vi "log analysis_gps.vi"() -> ()   [LabVIEW 2019] (continued)
normal 2 28.000000 0 0\trobot status\t224.454094\t106.289385\t8.223600\t-0.397359\t-0.581660\t162.070922\t0.000000\t0.000000\n\t\n15:40:00.3\tlog_raw\tgps_raw\t\tsystem status\tnormal 2 28.000000 0 0\trobot status\t224.454354\t106.289109\t8.223500\t-0.396354\t-0.583432\t162.070544\t0.000000\t0.000000\n\t\n15:40:00.8\tlog_raw\tgps_raw\t#INSPVAXA,USB3,0,49.0,FINESTEERING,2107,283218.850,02000000,471d,15824;INS_ALIGNMENT_COMPLETE,INS_RTKFIXED,37.37108791456,126.72336907619,8.2236,22.3000,0.0037,0.0083,-0.0011,-0.397325323,-0.588631877,287.932091771,0.2122,0.1575,0.2639,0.0344,0.0343,0.0312,0.0792,0.0802,5.0844,0f000005,0*75bb9db3\n\tsystem status\tnormal 2 28.000000 0 0\trobot status\t224.455009\t106.288943\t8.223600\t-0.397325\t-0.588632\t162.067908\t0.000000\t0.000000\n\t\n15:40:01.3\tlog_raw\tgps_raw\t#INSPVAXA,USB3,0,48.5,FINESTEERING,2107,283219.350,02000000,471d,15824;INS_ALIGNMENT_COMPLETE,INS_RTKFIXED,37.37108791216,126.72336907891,8.2235,22.3000,0.0033,0.0082,-0.0011,-0.397206354,-0.592415954,287.932797733,0.2122,0.1575,0.2639,0.0344,0.0343,0.0312,0.0792,0.0802,5.0858,0f000005,0*61ec993c\n\tsystem status\tnormal 2 28.000000 0 0\trobot status\t224.455250\t106.288677\t8.223500\t-0.397206\t-0.592416\t162.067202\t0.000000\t0.000000\n\t\n15:40:01.8\tlog_raw\tgps_raw\t#DUALANTENNAHEADINGA,USB3,0,48.5,FINESTEERING,2107,283219.800,02000000,d426,15824;INSUFFICIENT_OBS,NONE,-1.000000000,0.000000000,0.000000000,0.0,0.000000000,0.000000000,\"631T\",12,4,4,3,04,00,20,03*1f4b872e\n\tsystem status\tnormal 2 28.000000 0 0\trobot status\t224.455582\t106.288430\t8.223100\t-0.398043\t-0.597040\t162.064293\t0.000000\t0.000000\n\t\n15:40:02.3\tlog_raw\tgps_raw\t#INSPVAXA,USB3,0,49.5,FINESTEERING,2107,283220.350,02000000,471d,15824;INS_ALIGNMENT_COMPLETE,INS_RTKFIXED,37.37108790624,126.72336908505,8.2229,22.3000,0.0022,0.0079,-0.0019,-0.399821313,-0.599696922,287.937754794,0.2122,0.1575,0.2639,0.0344,0.0343,0.0312,0.0792,0.0802,5.0871,0f000005,0*02520bc5\n\tsystem status\tnormal 2 28.000000 0 0\trobot status\t224.455794\t106.288020\t8.222900\t-0.399821\t-0.599697\t162.062245\t0.000000\t0.000000\n\t\n15:40:02.8\tlog_raw\tgps_raw\t#DUALANTENNAHEADINGA,USB3,0,49.5,FINESTEERING,2107,283220.800,02000000,d426,15824;INSUFFICIENT_OBS,NONE,-1.000000000,0.000000000,0.000000000,0.0,0.000000000,0.000000000,\"631T\",14,4,4,3,04,00,20,03*89ffa4d7\n\tsystem status\tnormal 2 28.000000 0 0\trobot status\t224.456145\t106.287761\t8.222900\t-0.400058\t-0.601408\t162.059931\t0.000000\t0.000000\n\t\n15:40:03.3\tlog_raw\tgps_raw\t#INSPVAXA,USB3,0,50.0,FINESTEERING,2107,283221.350,02000000,471d,15824;INS_ALIGNMENT_COMPLETE,INS_RTKFIXED,37.37108790285,126.72336908925,8.2228,22.3000,0.0035,0.0061,-0.0019,-0.399017543,-0.601198983,287.941471827,0.2122,0.1575,0.2639,0.0344,0.0343,0.0312,0.0792,0.0802,5.0886,0f000005,0*62ae3a3c\n\tsystem status\tnormal 2 28.000000 0 0\trobot status\t224.456166\t106.287643\t8.222800\t-0.399018\t-0.601199\t162.058528\t0.000000\t0.000000\n\t\n15:40:03.8\tlog_raw\tgps_raw\t#DUALANTENNAHEADINGA,USB3,0,50.0,FINESTEERING,2107,283221.800,02000000,d426,15824;INSUFFICIENT_OBS,NONE,-1.000000000,0.000000000,0.000000000,0.0,0.000000000,0.000000000,\"631T\",15,4,4,3,04,00,20,03*47e08abb\n\tsystem status\tnormal 2 28.000000 0 0\trobot status\t224.456082\t106.288102\t8.222400\t-0.398407\t-0.602014\t162.056223\t0.000000\t0.000000\n\t\n15:40:04.3\tlog_raw\tgps_raw\t#INSPVAXA,USB3,0,45.5,FINESTEERING,2107,283222.350,02000000,471d,15824;INS_ALIGNMENT_COMPLETE,INS_RTKFIXED,37.37108790796,126.72336908471,8.2224,22.3000,0.0048,0.0047,-0.0019,-0.398683572,-0.604525422,287.944164472,0.2123,0.1575,0.2638,0.0344,0.0343,0.0312,0.0792,0.0802,5.0901,0f000005,0*5070a156\n\tsystem status\tnormal 2 28.000000 0 0\trobot status\t224.455764\t106.288211\t8.222400\t-0.398684\t-0.604525\t162.055836\t0.000000\t0.000000\n\t\n15:40:04.8\tlog_raw\tgps_raw\t#DUALANTENNAHEADINGA,USB3,0,45.5,FINESTEERING,2107,283222.800,02000000,d426,15824;INSUFFICIENT_OBS,NONE,-1.000000000,0.000000000,0.000000000,0.0,0.000000000,0.000000000,\"631T\",14,4,4,3,04,00,20,03*8ce94816\n\tsystem status\tnormal 2 28.000000 0 0\trobot status\t224.455489\t106.288239\t8.222400\t-0.397979\t-0.605286\t162.052954\t0.000000\t0.000000\n\t\n15:40:05.3\tlog_raw\tgps_raw\t#INSPVAXA,USB3,0,50.0,FINESTEERING,2107,283223.350,02000000,471d,15824;INS_ALIGNMENT_COMPLETE,INS_RTKFIXED,37.37108790821,126.72336907660,8.2226,22.3000,0.0055,0.0030,-0.0018,-0.398800774,-0.606505226,287.948554602,0.2123,0.1575,0.2638,0.0344,0.0343,0.0312,0.0792,0.0802,5.0917,0f000005,0*2b7dac3f\n\tsystem status\tnormal 2 28.000000 0 0\trobot status\t224.455045\t106.288238\t8.222600\t-0.398801\t-0.606505\t162.051445\t0.000000\t0.000000\n\t\n15:40:05.8\tlog_raw\tgps_raw\t\tsystem status\tnormal 2 28.000000 0 0\trobot status\t224.454616\t106.288408\t8.223000\t-0.399540\t-0.605602\t162.051000\t0.000000\t0.000000\n\t\n15:40:06.3\tlog_raw\tgps_raw\t#DUALANTENNAHEADINGA,USB3,0,49.5,FINESTEERING,2107,283224.300,02000000,d426,15824;INSUFFICIENT_OBS,NONE,-1.000000000,0.000000000,0.000000000,0.0,0.000000000,0.000000000,\"631T\",16,4,4,3,04,00,20,03*04689537\n\tsystem status\tnormal 2 28.000000 0 0\trobot status\t224.454250\t106.288382\t8.223000\t-0.399365\t-0.605451\t162.052103\t0.000000\t0.000000\n\t\n15:40:06.8\tlog_raw\tgps_raw\t#INSPVAXA,USB3,0,49.5,FINESTEERING,2107,283224.850,02000000,471d,15824;INS_ALIGNMENT_COMPLETE,INS_RTKFIXED,37.37108790871,126.72336906996,8.2222,22.3000,0.0045,0.0021,-0.0033,-0.398675673,-0.605186622,287.948531011,0.2123,0.1575,0.2638,0.0344,0.0343,0.0312,0.0792,0.0802,5.0933,0f000005,0*5d419d28\n\tsystem status\tnormal 2 28.000000 0 0\trobot status\t224.454457\t106.288294\t8.222200\t-0.398676\t-0.605187\t162.051469\t0.000000\t0.000000\n\t\n15:40:07.3\tlog_raw\tgps_raw\t#INSPVAXA,USB3,0,47.0,FINESTEERING,2107,283225.350,02000000,471d,15824;INS_ALIGNMENT_COMPLETE,INS_RTKFIXED,37.37108790579,126.72336906833,8.2219,22.3000,0.0039,0.0019,-0.0038,-0.399713651,-0.605242342,287.947949852,0.2123,0.1575,0.2638,0.0344,0.0343,0.0312,0.0792,0.0802,5.0949,0f000005,0*a40dd195\n\tsystem status\tnormal 2 28.000000 0 0\trobot status\t224.454313\t106.287970\t8.221900\t-0.399714\t-0.605242\t162.052050\t0.000000\t0.000000\n\t\n15:40:07.8\tlog_raw\tgps_raw\t#INSPVAXA,USB3,0,47.0,FINESTEERING,2107,283225.850,02000000,471d,15824;INS_ALIGNMENT_COMPLETE,INS_RTKFIXED,37.37108794475,126.72336891478,8.2224,22.3000,0.0658,-0.1833,-0.0010,-0.392923625,-0.435798491,288.066022775,0.2123,0.1575,0.2638,0.0344,0.0343,0.0312,0.0792,0.0802,5.0949,0f000005,0*2ff36e63\n\tsystem status\tnormal 2 27.900000 0 0\trobot status\t224.440712\t106.292294\t8.222400\t-0.392924\t-0.435798\t161.933977\t0.180000\t0.055000\n\t\n15:40:08.3\tlog_raw\tgps_raw\t#INSPVAXA,USB3,0,49.0,FINESTEERING,2107,283226.350,02000000,471d,15824;INS_ALIGNMENT_COMPLETE,INS_RTKFIXED,37.37108844765,126.72336703725,8.2202,22.3000,0.1175,-0.3192,-0.0049,-0.452699232,-0.802169824,288.131784608,0.2162,0.1626,0.2698,0.0571,0.0479,0.0400,0.0831,0.0841,5.0965,0f000001,0*8912b163\n\tsystem status\tnormal 2 28.000000 0 0\trobot status\t224.274403\t106.348113\t8.220200\t-0.452699\t-0.802170\t161.868215\t0.327000\t-0.008000\n\t\n15:40:08.8\tlog_raw\tgps_raw\t\tsystem status\tnormal 2 28.000000 0 0\trobot status\t224.153734\t106.388805\t8.217000\t-0.710423\t-0.963431\t161.777362\t0.275000\t0.048000\n\t\n15:40:09.3\tlog_raw\tgps_raw\t#INSPVAXA,USB3,0,48.5,FINESTEERING,2107,283227.350,02000000,471d,15824;INS_ALIGNMENT_COMPLETE,INS_RTKFIXED,37.37108931483,126.72336395391,8.2149,22.3000,0.1129,-0.2937,-0.0022,-0.567222074,-1.168347253,288.238962529,0.2212,0.1749,0.2808,0.0651,0.0592,0.0471,0.0869,0.0878,5.0924,0f000001,0*8f246b52\n\tsystem status\tnormal 2 28.000000 0 0\trobot status\t224.001286\t106.444364\t8.214900\t-0.567222\t-1.168347\t161.761037\t0.292000\t0.057000\n\t\n15:40:09.8\tlog_raw\tgps_raw\t#INSPVAXA,USB3,0,48.5,FINESTEERING,2107,283227.850,02000000,471d,15824;INS_ALIGNMENT_COMPLETE,INS_RTKFIXED,37.37108976815,126.72336241064,8.2129,22.3000,0.1012,-0.2894,0.0009,-0.427491703,-1.215964317,288.177638677,0.2212,0.1749,0.2808,0.0651,0.0592,0.0471,0.0869,0.0878,5.0924,0f000001,0*ddfdf890\n\tsystem status\tnormal 2 27.900000 0 0\trobot status\t223.864586\t106.494679\t8.212900\t-0.427492\t-1.215964\t161.822361\t0.383000\t-0.102000\n\t\n15:40:10.3\tlog_raw\tgps_raw\t#INSPVAXA,USB3,0,43.5,FINESTEERING,2107,283228.350,02000000,471d,15824;INS_ALIGNMENT_COMPLETE,INS_RTKFIXED,37.37109022271,126.72336087108,8.2100,22.3000,0.0996,-0.2735,0.0003,-0.409798448,-1.329111694,287.820965193,0.2393,0.1944,0.2974,0.0761,0.0698,0.0531,0.0903,0.0914,5.0788,0f000001,0*ba2a3ea8\n\tsystem status\tnormal 2 27.900000 0 0\trobot status\t223.728214\t106.545132\t8.210000\t-0.409798\t-1.329112\t162.179035\t0.286000\t0.039000\n\t\n15:40:10.8\tlog_raw\tgps_raw\t#INSPVAXA,USB3,0,43.5,FINESTEERING,2107,283228.850,02000000,471d,15824;INS_ALIGNMENT_COMPLETE,INS_RTKFIXED,37.37109066362,126.72335936248,8.2065,22.3000,0.0986,-0.2652,0.0020,-0.598740198,-1.345095429,287.386151451,0.2393,0.1944,0.2974,0.0761,0.0698,0.0531,0.0903,0.0914,5.0788,0f000001,0*2e7dd81d\n\tsystem status\tnormal 2 27.900000 0 0\trobot status\t223.594584\t106.594070\t8.206500\t-0.598740\t-1.345095\t162.613849\t0.240000\t0.109000\n\t\n15:40:11.3\tlog_raw\tgps_raw\t#INSPVAXA,USB3,0,48.5,FINESTEERING,2107,283229.350,02000000,471d,15824;INS_ALIGNMENT_COMPLETE,INS_RTKFIXED,37.37109112291,126.72335786047,8.2034,22.3000,0.1037,-0.2722,0.0059,-0.580011682,-1.182180858,286.853066758,0.2680,0.2186,0.3192,0.0865,0.0782,0.0582,0.0931,0.0946,5.0540,0f000001,0*9b5ccdcf\n\tsystem status\tnormal 2 27.800000 0 0\trobot status\t223.461539\t106.645047\t8.203400\t-0.580012\t-1.182181\t163.146933\t0.284000\t0.047000\n\t\n15:40:11.8\tlog_raw\tgps_raw\t#INSPVAXA,USB3,0,48.5,FINESTEERING,2107,283229.850,02000000,471d,15824;INS_ALIGNMENT_COMPLETE,INS_RTKFIXED,37.37109159656,126.72335634766,8.2007,22.3000,0.0997,-0.2660,0.0048,-0.505114639,-1.253978500,286.329147717,0.2680,0.2186,0.3192,0.0865,0.0782,0.0582,0.0931,0.0946,5.0540,0f000001,0*b8c54619\n\tsystem status\tnormal 2 27.800000 0 0\trobot status\t223.327537\t106.697619\t8.200700\t-0.505115\t-1.253979\t163.670852\t0.201000\t0.152000\n\t\n15:40:12.3\tlog_raw\tgps_raw\t\tsystem status\tnormal 2 27.800000 0 0\trobot status\t223.205787\t106.745862\t8.197500\t-0.502623\t-1.292688\t164.218848\t0.298000\t0.019000\n\t\n15:40:12.8\tlog_raw\tgps_raw\t#INSPVAXA,USB3,0,48.5,FINESTEERING,2107,283230.850,02000000,471d,15824;INS_ALIGNMENT_COMPLETE,INS_RTKFIXED,37.37109255379,126.72335333433,8.1922,22.3000,0.1139,-0.2722,-0.0264,-0.549844601,-1.243677147,285.192352879,0.3030,0.2423,0.3452,0.0951,0.0845,0.0626,0.0951,0.0973,5.0218,0f000001,0*4712ada1\n\tsystem status\tnormal 2 27.700000 0 0\trobot status\t223.060621\t106.803864\t8.192200\t-0.549845\t-1.243677\t164.807647\t0.237000\t0.112000\n\t\n15:40:13.3\tlog_raw\tgps_raw\t\tsystem status\tnormal 2 27.800000 0 0\trobot status\t222.939771\t106.853141\t8.188200\t-0.588387\t-1.223015\t165.124564\t0.226000\t0.121000\n\t\n15:40:13.8\tlog_raw\tgps_raw\t#INSPVAXA,USB3,0,47.5,FINESTEERING,2107,283231.850,02000000,471d,15824;INS_ALIGNMENT_COMPLETE,INS_RTKFIXED,37.37109356016,126.72335031478,8.1824,22.3000,0.1080,-0.2773,-0.0065,-0.427440692,-1.278596031,284.403841092,0.3386,0.2620,0.3738,0.1014,0.0883,0.0663,0.0962,0.0993,4.9874,0f000001,0*03e37570\n\tsystem status\tnormal 2 27.900000 0 0\trobot status\t222.793154\t106.915562\t8.182400\t-0.427441\t-1.278596\t165.596159\t0.216000\t0.140000\n\t\n15:40:14.3\tlog_raw\tgps_raw\t\tsystem status\tnormal 2 27.900000 0 0\trobot status\t222.674508\t106.965363\t8.178200\t-0.397587\t-1.349561\t165.862378\t0.359000\t-0.071000\n\t\n15:40:14.8\tlog_raw\tgps_raw\t\tsystem status\tnormal 2 27.900000 0 0\trobot status\t222.542928\t107.019957\t8.172800\t-0.416047\t-1.243660\t166.159650\t0.279000\t0.039000\n\t\n15:40:15.3\tlog_raw\tgps_raw\t#INSPVAXA,USB3,0,48.5,FINESTEERING,2107,283233.350,02000000,471d,15824;INS_ALIGNMENT_COMPLETE,INS_RTKFIXED,37.37109506136,126.72334582781,8.1673,22.3000,0.1059,-0.2882,-0.0129,-0.399188016,-1.308966160,283.569134485,0.3953,0.2852,0.4320,0.1083,0.0909,0.0717,0.0969,0.1016,4.9362,0f000001,0*c0c0ad69\n\tsystem status\tnormal 2 27.900000 0 0\trobot status\t222.395706\t107.082183\t8.167300\t-0.399188\t-1.308966\t166.430866\t0.280000\t0.051000\n\t\n15:40:15.8\tlog_raw\tgps_raw\t#INSPVAXA,USB3,0,48.5,FINESTEERING,2107,283233.850,02000000,471d,15824;INS_ALIGNMENT_COMPLETE,INS_RTKFIXED,37.37109557748,126.72334434749,8.1612,22.3000,0.1020,-0.2689,-0.0118,-0.288207427,-1.260427493,283.382499321,0.3953,0.2852,0.4320,0.1083,0.0909,0.0717,0.0969,0.1016,4.9362,0f000001,0*9cae95f0\n\tsystem status\tnormal 2 27.900000 0 0\trobot status\t222.264581\t107.139468\t8.161200\t-0.288207\t-1.260427\t166.617501\t0.269000\t0.054000\n\t\n15:40:16.3\tlog_raw\tgps_raw\t#INSPVAXA,USB3,0,40.5,FINESTEERING,2107,283234.350,02000000,471d,15824;INS_ALIGNMENT_COMPLETE,INS_RTKFIXED,37.37109597071,126.72334335857,8.1556,22.3000,0.0926,-0.1801,-0.0168,-0.385399344,-0.992179167,283.170226692,0.4136,0.2904,0.4588,0.1097,0.0911,0.0735,0.0969,0.1021,4.9239,0f000001,0*8e2cf425\n\tsystem status\tnormal 2 27.900000 0 0\trobot status\t222.176984\t107.183113\t8.155600\t-0.385399\t-0.992179\t166.829773\t0.175000\t0.049000\n\t\n15:40:16.8\tlog_raw\tgps_raw\t\tsystem status\tnormal 2 27.900000 0 0\trobot status\t222.041325\t107.237168\t8.148500\t-0.223084\t-1.273652\t166.883018\t0.182000\t0.108000\n\t\n15:40:17.3\tlog_raw\tgps_raw\t#INSPVAXA,USB3,0,44.5,FINESTEERING,2107,283235.350,02000000,471d,15824;INS_ALIGNMENT_COMPLETE,INS_RTKFIXED,37.37109700062,126.72334017325,8.1414,22.3000,0.1228,-0.2164,-0.0234,-0.044307272,-1.163346566,282.981780278,0.4261,0.2932,0.4825,0.1104,0.0912,0.0747,0.0969,0.1023,4.9187,0f000001,0*f944742e\n\tsystem status\tnormal 2 27.900000 0 0\trobot status\t221.894834\t107.297424\t8.141400\t-0.044307\t-1.163347\t167.018220\t0.186000\t0.129000\n\t\n15:40:17.8\tlog_raw\tgps_raw\t#INSPVAXA,USB3,0,44.5,FINESTEERING,2107,283235.850,02000000,471d,15824;INS_ALIGNMENT_COMPLETE,INS_RTKFIXED,37.37109748848,126.72333864124,8.1345,22.3000,0.1343,-0.2501,-0.0261,0.047074074,-1.173722020,282.896627938,0.4261,0.2932,0.4825,0.1104,0.0912,0.0747,0.0969,0.1023,4.9187,0f000001,0*d201ba2d\n\tsystem status\tnormal 2 27.900000 0 0\trobot status\t221.759131\t107.351573\t8.134500\t0.047074\t-1.173722\t167.103372\t0.376000\t-0.123000\n\t\n15:40:18.3\tlog_raw\tgps_raw\t#INSPVAXA,USB3,0,49.0,FINESTEERING,2107,283236.350,02000000,471d,15824;INS_ALIGNMENT_COMPLETE,INS_RTKFIXED,37.37109796118,126.72333710973,8.1282,22.3000,0.1356,-0.2699,-0.0252,0.117707289,-1.086574547,282.783735366,0.4343,0.2946,0.5028,0.1112,0.0912,0.0756,0.0969,0.1025,4.9173,0f000001,0*2a8403f7\n\tsystem status\tnormal 2 27.900000 0 0\trobot status\t221.623472\t107.404039\t8.128200\t0.117707\t-1.086575\t167.216265\t0.368000\t-0.094000\n\t\n15:40:18.8\tlog_raw\tgps_raw\t#INSPVAXA,USB3,0,49.0,FINESTEERING,2107,283236.850,02000000,471d,15824;INS_ALIGNMENT_COMPLETE,INS_RTKFIXED,37.37109843766,126.72333556115,8.1224,22.3000,0.1364,-0.2752,-0.0170,0.206554754,-1.115785286,282.668706587,0.4343,0.2946,0.5028,0.1112,0.0912,0.0756,0.0969,0.1025,4.9173,0f000001,0*f32b757d\n\tsystem status\tnormal 2 27.900000 0 0\trobot status\t221.486302\t107.456924\t8.122400\t0.206555\t-1.115785\t167.331293\t0.349000\t-0.069000\n\t\n15:40:19.3\tlog_raw\tgps_raw\t#INSPVAXA,USB3,0,50.0,FINESTEERING,2107,283237.350,02000000,471d,15824;INS_ALIGNMENT_COMPLETE,INS_RTKFIXED,37.37109889709,126.72333402852,8.1172,22.3000,0.1302,-0.2622,-0.0159,0.272964655,-0.969484685,282.581344879,0.4398,0.2952,0.5196,0.1116,0.0914,0.0761,0.0969,0.1026,4.9185,0f000001,0*477c8ced\n\tsystem status\tnormal 2 27.900000 0 0\trobot status\t221.350544\t107.507918\t8.117200\t0.272965\t-0.969485\t167.418655\t0.348000\t-0.074000\n\t\n15:40:19.8\tlog_raw\tgps_raw\t#INSPVAXA,USB3,0,50.0,FINESTEERING,2107,283237.850,02000000,471d,15824;INS_ALIGNMENT_COMPLETE,INS_RTKFIXED,37.37109934536,126.72333248224,8.1121,22.3000,0.1280,-0.2768,-0.0138,0.258054665,-1.050370160,282.484517090,0.4398,0.2952,0.5196,0.1116,0.0914,0.0761,0.0969,0.1026,4.9185,0f000001,0*cd2f787f\n\tsystem status\tnormal 2 27.900000 0 0\trobot status\t221.213577\t107.557672\t8.112100\t0.258055\t-1.050370\t167.515483\t0.336000\t-0.058000\n\t\n15:40:20.3\tlog_raw\tgps_raw\t#INSPVAXA,USB3,0,51.5,FINESTEERING,2107,283238.350,02000000,471d,15824;INS_ALIGNMENT_COMPLETE,INS_RTKFIXED,37.37109977982,126.72333093578,8.1070,22.3000,0.1223,-0.2761,-0.0142,0.234355283,-1.035161651,282.464995705,0.4436,0.2955,0.5329,0.1118,0.0916,0.0764,0.0970,0.1026,4.9197,0f000001,0*b2aac9f1\n\tsystem status\tnormal 2 27.900000 0 0\trobot status\t221.076594\t107.605894\t8.107000\t0.234355\t-1.035162\t167.535004\t0.373000\t-0.110000\n\t\n15:40:20.8\tlog_raw\tgps_raw\t#INSPVAXA,USB3,0,51.5,FINESTEERING,2107,283238.850,02000000,471d,15824;INS_ALIGNMENT_COMPLETE,INS_RTKFIXED,37.37110022418,126.72332937535,8.1011,22.3000,0.1168,-0.2700,-0.0206,0.387659618,-1.151934969,282.487408850,0.4436,0.2955,0.5329,0.1118,0.0916,0.0764,0.0970,0.1026,4.9197,0f000001,0*91317f18\n\tsystem status\tnormal 2 28.000000 0 0\trobot status\t220.938374\t107.655215\t8.101100\t0.387660\t-1.151935\t167.512591\t0.298000\t-0.003000\n\t\n15:40:21.3\tlog_raw\tgps_raw\t#INSPVAXA,USB3,0,49.0,FINESTEERING,2107,283239.350,02000000,471d,15824;INS_ALIGNMENT_COMPLETE,INS_RTKFIXED,37.37110063479,126.72332783214,8.0954,22.3000,0.1184,-0.2911,-0.0146,0.524963643,-1.181982568,282.530354498,0.4459,0.2956,0.5431,0.1123,0.0918,0.0765,0.0970,0.1026,4.9196,0f000001,0*aac06e63\n\tsystem status\tnormal 2 27.900000 0 0\trobot status\t220.801679\t107.700790\t8.095400\t0.524964\t-1.181983\t167.469646\t0.299000\t0.005000\n\t\n15:40:21.8\tlog_raw\tgps_raw\t#INSPVAXA,USB3,0,49.0,FINESTEERING,2107,283239.850,02000000,471d,15824;INS_ALIGNMENT_COMPLETE,INS_RTKFIXED,37.37110101931,126.72332626888,8.0896,22.3000,0.1173,-0.2983,-0.0228,0.347504334,-1.218326130,282.608811447,0.4459,0.2956,0.5431,0.1123,0.0918,0.0765,0.0970,0.1026,4.9196,0f000001,0*aaab564a\n\tsystem status\tnormal 2 27.900000 0 0\trobot status\t220.663208\t107.743470\t8.089600\t0.347504\t-1.218326\t167.391189\t0.313000\t-0.016000\n\t\n15:40:22.3\tlog_raw\tgps_raw\t#INSPVAXA,USB3,0,49.5,FINESTEERING,2107,283240.350,02000000,471d,15824;INS_ALIGNMENT_COMPLETE,INS_RTKFIXED,37.37110139226,126.72332471479,8.0839,22.3000,0.1052,-0.2558,-0.0218,0.111794667,-1.199195640,282.711507437,0.4475,0.2957,0.5507,0.1121,0.0921,0.0765,0.0971,0.1026,4.9179,0f000001,0*067ad1f3\n\tsystem status\tnormal 2 28.000000 0 0\trobot status\t220.525549\t107.784865\t8.083900\t0.111795\t-1.199196\t167.288493\t0.283000\t-0.006000\n\t\n15:40:22.8\tlog_raw\tgps_raw\t#INSPVAXA,USB3,0,49.5,FINESTEERING,2107,283240.850,02000000,471d,15824;INS_ALIGNMENT_COMPLETE,INS_RTKFIXED,37.37110178506,126.72332315971,8.0792,22.3000,0.1224,-0.2728,-0.0239,0.192223977,-1.143692824,282.808782455,0.4475,0.2957,0.5507,0.1121,0.0921,0.0765,0.0971,0.1026,4.9179,0f000001,0*4c669a89\n\tsystem status\tnormal 2 27.900000 0 0\trobot status\t220.387802\t107.828463\t8.079200\t0.192224\t-1.143693\t167.191218\t0.304000\t-0.009000\n\t\n15:40:23.3\tlog_raw\tgps_raw\t#INSPVAXA,USB3,0,46.0,FINESTEERING,2107,283241.350,02000000,471d,15824;INS_ALIGNMENT_COMPLETE,INS_RTKFIXED,37.37110216671,126.72332169027,8.0740,22.3000,0.1256,-0.2749,-0.0357,0.303484738,-0.991943095,282.906858014,0.4483,0.2959,0.5565,0.1130,0.0923,0.0766,0.0971,0.1026,4.9153,0f000001,0*4b7c655e\n\tsystem status\tnormal 2 27.900000 0 0\trobot status\t220.257642\t107.870824\t8.074000\t0.303485\t-0.991943\t167.093142\t0.302000\t-0.011000\n\t\n15:40:23.8\tlog_raw\tgps_raw\t\tsystem status\tnormal 2 28.000000 0 0\trobot status\t220.122992\t107.913992\t8.068800\t0.222586\t-0.858858\t166.913815\t0.296000\t-0.018000\n\t\n15:40:24.3\tlog_raw\tgps_raw\t#INSPVAXA,USB3,0,49.5,FINESTEERING,2107,283242.350,02000000,471d,15824;INS_ALIGNMENT_COMPLETE,INS_RTKFIXED,37.37110294523,126.72331868826,8.0634,22.3000,0.1292,-0.2803,-0.0380,0.123672513,-0.689289621,283.242371954,0.4492,0.2961,0.5604,0.1137,0.0926,0.0766,0.0971,0.1026,4.9113,0f000001,0*f9b22440\n\tsystem status\tnormal 2 27.900000 0 0\trobot status\t219.991729\t107.957235\t8.063400\t0.123673\t-0.689290\t166.757628\t0.298000\t-0.030000\n\t\n15:40:24.8\tlog_raw\tgps_raw\t#INSPVAXA,USB3,0,49.5,FINESTEERING,2107,283242.850,02000000,471d,15824;INS_ALIGNMENT_COMPLETE,INS_RTKFIXED,37.37110335770,126.72331719520,8.0593,22.3000,0.1255,-0.2698,-0.0380,0.121355626,-0.605377000,283.439898811,0.4492,0.2961,0.5604,0.1137,0.0926,0.0766,0.0971,0.1026,4.9113,0f000001,0*de8b7806\n\tsystem status\tnormal 2 27.900000 0 0\trobot status\t219.859476\t108.003016\t8.059300\t0.121356\t-0.605377\t166.560101\t0.296000\t-0.017000\n\t\n15:40:25.3\tlog_raw\tgps_raw\t\tsystem status\tnormal 2 27.900000 0 0\trobot status\t219.719105\t108.051606\t8.055100\t0.093618\t-0.577412\t166.343650\t0.303000\t-0.020000\n\t\n15:40:25.8\tlog_raw\tgps_raw\t\tsystem status\tnormal 2 28.000000 0 0\trobot status\t219.581090\t108.101532\t8.050400\t0.152820\t-0.756996\t166.118553\t0.299000\t-0.020000\n\t\n15:40:26.3\tlog_raw\tgps_raw\t#INSPVAXA,USB3,0,49.0,FINESTEERING,2107,283244.350,02008000,471d,15824;INS_ALIGNMENT_COMPLETE,INS_RTKFIXED,37.37110468880,126.72331252353,8.0457,22.3000,0.1303,-0.2564,-0.0224,0.139221287,-0.844011919,284.159794533,0.4505,0.2963,0.5646,0.1137,0.0927,0.0766,0.0971,0.1025,4.8983,0f000001,0*7deeba4a\n\tsystem status\tnormal 2 28.000000 0 0\trobot status\t219.445667\t108.150759\t8.045700\t0.139221\t-0.844012\t165.840205\t0.283000\t-0.044000\n\t\n15:40:26.8\tlog_raw\tgps_raw\t#INSPVAXA,USB3,0,49.0,FINESTEERING,2107,283244.850,02008000,471d,15824;INS_ALIGNMENT_COMPLETE,INS_RTKFIXED,37.37110513730,126.72331104111,8.0417,22.3000,0.1309,-0.2685,-0.0243,0.209910171,-0.848689827,284.605167035,0.4505,0.2963,0.5646,0.1137,0.0927,0.0766,0.0971,0.1025,4.8983,0f000001,0*e4fb8053\n\tsystem status\tnormal 2 27.900000 0 0\trobot status\t219.314357\t108.200539\t8.041700\t0.209910\t-0.848690\t165.394833\t0.220000\t-0.144000\n\t\n15:40:27.3\tlog_raw\tgps_raw\t#INSPVAXA,USB3,0,50.0,FINESTEERING,2107,283245.350,02008000,471d,15824;INS_ALIGNMENT_COMPLETE,INS_RTKFIXED,37.37110557782,126.72330954830,8.0387,22.3000,0.1426,-0.2572,-0.0360,0.139361200,-0.921723778,285.121059969,0.4506,0.2964,0.5656,0.1138,0.0927,0.0767,0.0971,0.1024,4.8921,0f000001,0*fcb5f941\n\tsystem status\tnormal 2 27.900000 0 0\trobot status\t219.182126\t108.249433\t8.038700\t0.139361\t-0.921724\t164.878940\t0.304000\t0.001000\n\t\n15:40:27.8\tlog_raw\tgps_raw\t\tsystem status\tnormal 2 27.900000 0 0\trobot status\t219.049410\t108.299799\t8.035500\t0.171858\t-0.957026\t164.246816\t0.249000\t-0.096000\n\t\n15:40:28.3\tlog_raw\tgps_raw\t#INSPVAXA,USB3,0,48.5,FINESTEERING,2107,283246.350,02008000,471d,15824;INS_ALIGNMENT_COMPLETE,INS_RTKFIXED,37.37110650296,126.72330657394,8.0329,22.3000,0.1463,-0.2502,-0.0217,0.213692795,-0.911589097,286.397564613,0.4505,0.2965,0.5663,0.1141,0.0927,0.0768,0.0971,0.1023,4.8873,0f000001,0*feddfe3b\n\tsystem status\tnormal 2 27.900000 0 0\trobot status\t218.918662\t108.352116\t8.032900\t0.213693\t-0.911589\t163.602435\t0.285000\t-0.026000\n\t\n15:40:28.8\tlog_raw\tgps_raw\t#INSPVAXA,USB3,0,48.5,FINESTEERING,2107,283246.850,02008000,471d,15824;INS_ALIGNMENT_COMPLETE,INS_RTKFIXED,37.37110698644,126.72330510005,8.0315,22.3000,0.1343,-0.2488,-0.0293,0.310721762,-0.889438345,287.090761589,0.4505,0.2965,0.5663,0.1141,0.0927,0.0768,0.0971,0.1023,4.8873,0f000001,0*ee8d45a4\n\tsystem status\tnormal 2 27.800000 0 0\trobot status\t218.788107\t108.405779\t8.031500\t0.310722\t-0.889438\t162.909238\t0.254000\t-0.086000\n\t\n15:40:29.3\tlog_raw\tgps_raw\t#INSPVAXA,USB3,0,47.0,FINESTEERING,2107,283247.350,02008000,471d,15824;INS_ALIGNMENT_COMPLETE,INS_RTKFIXED,37.37110746549,126.72330361825,8.0305,22.3000,0.1318,-0.2455,-0.0310,0.265513660,-1.003037989,287.732787222,0.4503,0.2965,0.5665,0.1141,0.0927,0.0768,0.0970,0.1023,4.8832,0f000001,0*16257acc\n\tsystem status\tnormal 2 27.800000 0 0\trobot status\t218.656852\t108.458949\t8.030500\t0.265514\t-1.003038\t162.267213\t0.293000\t-0.017000\n\t\n15:40:29.8\tlog_raw\tgps_raw\t\tsystem status\tnormal 2 27.900000 0 0\trobot status\t218.527453\t108.511501\t8.030600\t0.143674\t-1.011536\t161.686913\t0.270000\t-0.063000\n\t\n15:40:30.3\tlog_raw\tgps_raw\t#INSPVAXA,USB3,0,51.5,FINESTEERING,2107,283248.350,02008000,471d,15824;INS_ALIGNMENT_COMPLETE,INS_RTKFIXED,37.37110841164,126.72330070273,8.0292,22.3000,0.1212,-0.2566,-0.0210,0.033040840,-0.857112226,288.813321277,0.4501,0.2965,0.5666,0.1141,0.0927,0.0770,0.0970,0.1022,4.8803,0f000001,0*d8465b23\n\tsystem status\tnormal 2 27.900000 0 0\trobot status\t218.398600\t108.563964\t8.029200\t0.033041\t-0.857112\t161.186679\t0.321000\t0.015000\n\t\n15:40:30.8\tlog_raw\tgps_raw\t\tsystem status\tnormal 2 27.900000 0 0\trobot status\t218.268593\t108.617778\t8.027300\t0.041770\t-0.809439\t160.804701\t0.252000\t-0.085000\n\t\n15:40:31.3\tlog_raw\tgps_raw\t\tsystem status\tnormal 2 27.900000 0 0\trobot status\t218.140921\t108.672728\t8.026700\t0.114502\t-0.661479\t160.471237\t0.255000\t-0.082000\n\t\n15:40:31.8\tlog_raw\tgps_raw\t#INSPVAXA,USB3,0,48.5,FINESTEERING,2107,283249.850,02008000,471d,15824;INS_ALIGNMENT_COMPLETE,INS_RTKFIXED,37.37110988356,126.72329635950,8.0261,22.3000,0.1256,-0.2402,-0.0147,0.060845598,-0.557595115,289.806680124,0.4499,0.2965,0.5665,0.1144,0.0927,0.0771,0.0970,0.1022,4.8781,0f000001,0*763984e0\n\tsystem status\tnormal 2 27.900000 0 0\trobot status\t218.013884\t108.727334\t8.026100\t0.060846\t-0.557595\t160.193320\t0.300000\t0.000000\n\t\n15:40:32.3\tlog_raw\tgps_raw\t#INSPVAXA,USB3,0,49.5,FINESTEERING,2107,283250.350,02000000,471d,15824;INS_ALIGNMENT_COMPLETE,INS_RTKFIXED,37.37111038564,126.72329491003,8.0267,22.3000,0.1228,-0.2382,-0.0157,-0.018569181,-0.488431655,290.019315132,0.4500,0.2966,0.5665,0.1143,0.0928,0.0772,0.0970,0.1022,4.8762,0f000001,0*c58162f6\n\tsystem status\tnormal 2 27.900000 0 0\trobot status\t217.885492\t108.783061\t8.026700\t-0.018569\t-0.488432\t159.980685\t0.279000\t-0.024000\n\t\n15:40:32.8\tlog_raw\tgps_raw\t\tsystem status\tnormal 2 27.900000 0 0\trobot status\t217.756803\t108.839181\t8.027900\t-0.125763\t-0.589533\t159.804053\t0.308000\t0.006000\n\t\n15:40:33.3\tlog_raw\tgps_raw\t\tsystem status\tnormal 2 28.000000 0 0\trobot status\t217.632707\t108.894799\t8.030000\t-0.101173\t-0.661853\t159.647625\t0.298000\t0.013000\n\t\n15:40:33.8\tlog_raw\tgps_raw\t#INSPVAXA,USB3,0,49.5,FINESTEERING,2107,283251.850,02000000,471d,15824;INS_ALIGNMENT_COMPLETE,INS_RTKFIXED,37.37111192959,126.72329056644,8.0317,22.3000,0.1243,-0.2388,-0.0145,-0.052610032,-0.761049634,290.503776347,0.4499,0.2966,0.5666,0.1142,0.0928,0.0773,0.0970,0.1021,4.8746,0f000001,0*ba4c3e6a\n\tsystem status\tnormal 2 28.000000 0 0\trobot status\t217.500744\t108.954426\t8.031700\t-0.052610\t-0.761050\t159.496224\t0.301000\t0.009000\n\t\n15:40:34.3\tlog_raw\tgps_raw\t#INSPVAXA,USB3,0,49.5,FINESTEERING,2107,283252.350,02000000,471d,15824;INS_ALIGNMENT_COMPLETE,INS_RTKFIXED,37.37111241968,126.72328920118,8.0341,22.3000,0.1282,-0.2523,-0.0162,-0.150683297,-0.978077835,290.683925037,0.4496,0.2967,0.5667,0.1142,0.0928,0.0774,0.0970,0.1021,4.8737,0f000001,0*23232e95\n\tsystem status\tnormal 2 27.900000 0 0\trobot status\t217.379811\t109.008821\t8.034100\t-0.150683\t-0.978078\t159.316075\t0.296000\t0.003000\n\t\n15:40:34.8\tlog_raw\tgps_raw\t\tsystem status\tnormal 2 27.900000 0 0\trobot status\t217.248099\t109.068468\t8.037000\t-0.197003\t-1.127011\t159.182870\t0.164000\t-0.022000\n\t\n15:40:35.3\tlog_raw\tgps_raw\t\tsystem status\tnormal 2 28.000000 0 0\trobot status\t217.148157\t109.115317\t8.038600\t-0.238983\t-1.099526\t159.082533\t0.289000\t0.000000\n\t\n15:40:35.8\tlog_raw\tgps_raw\t#INSPVAXA,USB3,0,50.0,FINESTEERING,2107,283253.850,02000000,471d,15824;INS_ALIGNMENT_COMPLETE,INS_RTKFIXED,37.37111392592,126.72328504795,8.0397,22.3000,0.1448,-0.2935,-0.0163,-0.197937020,-0.955376116,291.000430762,0.4494,0.2968,0.5669,0.1142,0.0929,0.0775,0.0970,0.1021,4.8734,0f000001,0*886ef4ee\n\tsystem status\tnormal 2 27.900000 0 0\trobot status\t217.011925\t109.176000\t8.039700\t-0.197937\t-0.955376\t158.999569\t0.319000\t-0.010000\n\t\n15:40:36.3\tlog_raw\tgps_raw\t\tsystem status\tnormal 2 27.900000 0 0\trobot status\t216.883247\t109.235889\t8.041500\t-0.197838\t-0.952972\t158.940609\t0.283000\t0.009000\n\t\n15:40:36.8\tlog_raw\tgps_raw\t\tsystem status\tnormal 2 27.900000 0 0\trobot status\t216.748752\t109.298652\t8.043700\t-0.269231\t-0.952303\t158.957919\t0.257000\t0.073000\n\t\n15:40:37.3\tlog_raw\tgps_raw\t\tsystem status\tnormal 2 27.900000 0 0\trobot status\t216.617232\t109.359943\t8.045200\t-0.202537\t-1.067653\t159.099182\t0.196000\t0.143000\n\t\n15:40:37.8\tlog_raw\tgps_raw\t\tsystem status\tnormal 2 27.900000 0 0\trobot status\t216.483089\t109.420918\t8.047500\t-0.134121\t-1.336250\t159.348626\t0.254000\t0.083000\n\t\n15:40:38.3\tlog_raw\tgps_raw\t#INSPVAXA,USB3,0,47.0,FINESTEERING,2107,283256.350,02000000,471d,15824;INS_ALIGNMENT_COMPLETE,INS_RTKFIXED,37.37111667800,126.72327759739,8.0487,22.3000,0.1131,-0.2631,-0.0127,-0.014268903,-1.510864451,290.200992248,0.4483,0.2970,0.5675,0.1142,0.0929,0.0778,0.0970,0.1021,4.8754,0f000001,0*3c5e786f\n\tsystem status\tnormal 2 27.800000 0 0\trobot status\t216.351967\t109.481456\t8.048700\t-0.014269\t-1.510864\t159.799008\t0.298000\t0.023000\n\t\n15:40:38.8\tlog_raw\tgps_raw\t\tsystem status\tnormal 2 27.800000 0 0\trobot status\t216.220657\t109.540064\t8.049100\t-0.119900\t-1.537133\t160.334398\t0.186000\t0.193000\n\t\n15:40:39.3\tlog_raw\tgps_raw\t\tsystem status\tnormal 2 27.800000 0 0\trobot status\t216.089003\t109.598692\t8.048400\t-0.093820\t-1.306197\t160.795485\t0.256000\t0.091000\n\t\n15:40:39.8\tlog_raw\tgps_raw\t\tsystem status\tnormal 2 27.800000 0 0\trobot status\t215.956601\t109.656931\t8.047000\t-0.019215\t-1.150225\t161.440777\t0.220000\t0.139000\n\t\n15:40:40.3\tlog_raw\tgps_raw\t\tsystem status\tnormal 2 27.800000 0 0\trobot status\t215.824837\t109.713079\t8.045700\t0.001489\t-1.057476\t162.001220\t0.273000\t0.049000\n\t\n15:40:40.8\tlog_raw\tgps_raw\t\tsystem status\tnormal 2 27.800000 0 0\trobot status\t215.690317\t109.768335\t8.045000\t-0.029547\t-1.094838\t162.443087\t0.233000\t0.108000\n\t\n15:40:41.3\tlog_raw\tgps_raw\t\tsystem status\tnormal 2 27.800000 0 0\trobot status\t215.555584\t109.823560\t8.044700\t-0.032872\t-1.159908\t162.901449\t0.350000\t-0.056000\n\t\n15:40:41.8\tlog_raw\tgps_raw\t\tsystem status\tnormal 2 27.800000 0 0\trobot status\t215.423293\t109.878083\t8.045400\t0.058847\t-1.225580\t163.287253\t0.331000\t-0.033000\n\t\n15:40:42.3\tlog_raw\tgps_raw\t\tsystem status\tnormal 2 27.800000 0 0\trobot status\t215.290908\t109.931352\t8.044700\t0.101525\t-1.216890\t163.536721\t0.264000\t0.047000\n\t\n15:40:42.8\tlog_raw\tgps_raw\t\tsystem status\tnormal 2 27.800000 0 0\trobot status\t215.156345\t109.983735\t8.043900\t0.020360\t-1.127078\t163.761724\t0.364000\t-0.093000\n\t\n15:40:43.3\tlog_raw\tgps_raw\t\tsystem status\tnormal 2 27.900000 0 0\trobot status\t215.021016\t110.036141\t8.043100\t-0.109689\t-1.073067\t163.912794\t0.351000\t-0.079000\n\t\n15:40:43.8\tlog_raw\tgps_raw\t\tsystem status\tnormal 2 27.900000 0 0\trobot status\t214.887094\t110.088591\t8.041700\t-0.164860\t-1.083253\t163.998199\t0.342000\t-0.056000\n\t\n15:40:44.3\tlog_raw\tgps_raw\t\tsystem status\tnormal 2 27.900000 0 0\trobot status\t214.752428\t110.142002\t8.041100\t-0.119096\t-1.063202\t164.023642\t0.332000\t-0.056000\n\t\n15:40:44.9\tlog_raw\tgps_raw\t\tsystem status\tnormal 2 27.900000 0 0\trobot status\t214.617455\t110.195495\t8.041800\t-0.119936\t-1.092491\t163.931808\t0.366000\t-0.103000\n\t\n15:40:45.4\tlog_raw\tgps_raw\t\tsystem status\tnormal 2 27.900000 0 0\trobot status\t214.485862\t110.248547\t8.041500\t-0.060549\t-1.081685\t163.903712\t0.293000\t-0.001000\n\t\n15:40:45.9\tlog_raw\tgps_raw\t\tsystem status\tnormal 2 27.900000 0 0\trobot status\t214.351476\t110.302605\t8.039900\t-0.112881\t-1.015686\t163.825151\t0.271000\t0.023000\n\t\n15:40:46.4\tlog_raw\tgps_raw\t\tsystem status\tnormal 2 27.900000 0 0\trobot status\t214.215520\t110.354999\t8.037100\t-0.237897\t-1.027372\t163.751447\t0.311000\t-0.011000\n\t\n15:40:46.9\tlog_raw\tgps_raw\t\tsystem status\tnormal 2 28.000000 0 0\trobot status\t214.083708\t110.406068\t8.035500\t-0.369244\t-0.964821\t163.739646\t0.308000\t-0.008000\n\t\n15:40:47.4\tlog_raw\tgps_raw\t\tsystem status\tnormal 2 27.900000 0 0\trobot status\t213.947858\t110.460257\t8.034800\t-0.353293\t-0.984714\t163.656974\t0.287000\t-0.004000\n\t\n15:40:47.9\tlog_raw\tgps_raw\t\tsystem status\tnormal 2 27.900000 0 0\trobot status\t213.813576\t110.514896\t8.035100\t-0.315479\t-0.958573\t163.628671\t0.256000\t0.062000\n\t\n15:40:48.4\tlog_raw\tgps_raw\t\tsystem status\tnormal 2 27.900000 0 0\trobot status\t213.680292\t110.566682\t8.035400\t-0.459086\t-0.833565\t163.542632\t0.363000\t-0.087000\n\t\n15:40:48.9\tlog_raw\tgps_raw\t\tsystem status\tnormal 2 27.900000 0 0\trobot status\t213.547610\t110.619462\t8.035900\t-0.413342\t-0.817768\t163.512122\t0.267000\t0.054000\n\t\n15:40:49.4\tlog_raw\tgps_raw\t\tsystem status\tnormal 2 27.900000 0 0\trobot status\t213.410653\t110.674109\t8.032900\t-0.389935\t-0.910065\t163.463731\t0.271000\t0.037000\n\t\n15:40:49.9\tlog_raw\tgps_raw\t\tsystem status\tnormal 2 27.900000 0 0\trobot status\t213.274252\t110.728041\t8.029700\t-0.452287\t-0.952096\t163.492789\t0.372000\t-0.095000\n\t\n15:40:50.4\tlog_raw\tgps_raw\t\tsystem status\tnormal 2 27.900000 0 0\trobot status\t213.139807\t110.780103\t8.028400\t-0.595437\t-0.961919\t163.551753\t0.296000\t0.016000\n\t\n15:40:50.9\tlog_raw\tgps_raw\t\tsystem status\tnormal 2 27.900000 0 0\trobot status\t213.007852\t110.831326\t8.026600\t-0.638166\t-0.992979\t163.689570\t0.294000\t0.013000\n\t\n15:40:51.4\tlog_raw\tgps_raw\t\tsystem status\tnormal 2 27.900000 0 0\trobot status\t212.870931\t110.883643\t8.022700\t-0.608918\t-1.002385\t163.823433\t0.283000\t0.023000\n\t\n15:40:51.9\tlog_raw\tgps_raw\t\tsystem status\tnormal 2 27.900000 0 0\trobot status\t212.734729\t110.935381\t8.018300\t-0.646845\t-0.891660\t163.908673\t0.334000\t-0.044000\n\t\n15:40:52.4\tlog_raw\tgps_raw\t\tsystem status\tnormal 2 27.900000 0 0\trobot status\t212.600747\t110.986202\t8.015300\t-0.669070\t-0.863720\t164.032580\t0.278000\t0.047000\n\t\n15:40:52.9\tlog_raw\tgps_raw\t\tsystem status\tnormal 2 27.900000 0 0\trobot status\t212.466131\t111.036735\t8.012100\t-0.729278\t-0.933955\t164.116412\t0.364000\t-0.088000\n\t\n15:40:53.4\tlog_raw\tgps_raw\t\tsystem status\tnormal 2 27.900000 0 0\trobot status\t212.329648\t111.086450\t8.009500\t-0.956979\t-0.949059\t164.216816\t0.359000\t-0.082000\n\t\n15:40:53.9\tlog_raw\tgps_raw\t\tsystem status\tnormal 2 27.900000 0 0\trobot status\t212.241082\t111.123844\t8.008300\t-0.972595\t-0.720450\t164.489490\t0.368000\t-0.031000\n\t\n15:40:54.4\tlog_raw\tgps_raw\t\tsystem status\tnormal 2 27.900000 0 0\trobot status\t212.102499\t111.173835\t8.005600\t-0.915387\t-0.756548\t164.601815\t0.258000\t0.037000\n\t\n15:40:54.9\tlog_raw\tgps_raw\t\tsystem status\tnormal 2 27.900000 0 0\trobot status\t211.965459\t111.221778\t8.002300\t-0.893423\t-0.725366\t164.719924\t0.234000\t0.089000\n\t\n15:40:55.4\tlog_raw\tgps_raw\t\tsystem status\tnormal 2 27.900000 0 0\trobot status\t211.831724\t111.270180\t8.000500\t-0.773057\t-0.648751\t164.828548\t0.248000\t0.076000\n\t\n15:40:55.9\tlog_raw\tgps_raw\t\tsystem status\tnormal 2 27.900000 0 0\trobot status\t211.700737\t111.317887\t7.999900\t-0.741179\t-0.600048\t165.022857\t0.243000\t0.089000\n\t\n15:40:56.4\tlog_raw\tgps_raw\t\tsystem status\tnormal 2 27.900000 0 0\trobot status\t211.569532\t111.365832\t7.999200\t-0.654123\t-0.551574\t165.161608\t0.424000\t-0.189000\n\t\n15:40:56.9\tlog_raw\tgps_raw\t\tsystem status\tnormal 2 27.900000 0 0\trobot status\t211.435334\t111.413612\t7.998900\t-0.655614\t-0.616450\t165.232482\t0.254000\t0.080000\n\t\n15:40:57.4\tlog_raw\tgps_raw\t\tsystem status\tnormal 2 27.900000 0 0\trobot status\t211.301894\t111.460655\t7.998300\t-0.554121\t-0.665582\t165.357637\t0.354000\t-0.076000\n\t\n15:40:57.9\tlog_raw\tgps_raw\t\tsystem status\tnormal 2 27.900000 0 0\trobot status\t211.170223\t111.505749\t7.997400\t-0.534661\t-0.759469\t165.459316\t0.345000\t-0.074000\n\t\n15:40:58.4\tlog_raw\tgps_raw\t\tsystem status\tnormal 2 27.900000 0 0\trobot status\t211.034516\t111.551520\t7.996500\t-0.554460\t-0.875450\t165.546133\t0.332000\t-0.052000\n\t\n15:40:58.9\tlog_raw\tgps_raw\t#INSPVAXA,USB3,0,44.0,FINESTEERING,2107,283276.900,02000000,471d,15824;INS_ALIGNMENT_COMPLETE,INS_RTKFIXED,37.37113577898,126.72321589270,7.9963,22.3000,0.1042,-0.2583,-0.0142,-0.525742005,-1.010949392,284.316907769,0.4477,0.2970,0.5693,0.1141,0.0929,0.0780,0.0969,0.1021,4.9003,0f000001,0*b42fff2f\n\tsystem status\tnormal 2 27.900000 0 0\trobot status\t210.886266\t111.601510\t7.996300\t-0.525742\t-1.010949\t165.683092\t0.212000\t0.124000\n\t\n15:40:59.4\tlog_raw\tgps_raw\t\tsystem status\tnormal 2 27.900000 0 0\trobot status\t210.768424\t111.641632\t7.996400\t-0.498952\t-0.902878\t165.766110\t0.234000\t0.086000\n\t\n15:40:59.9\tlog_raw\tgps_raw\t#INSPVAXA,USB3,0,47.5,FINESTEERING,2107,283277.900,02000000,471d,15824;INS_ALIGNMENT_COMPLETE,INS_RTKFIXED,37.37113658418,126.72321294940,7.9963,22.3000,0.0900,-0.2507,-0.0130,-0.397975122,-0.687807065,284.132829935,0.4476,0.2970,0.5692,0.1141,0.0929,0.0780,0.0969,0.1021,4.9017,0f000001,0*e88e7117\n\tsystem status\tnormal 2 27.900000 0 0\trobot status\t210.625554\t111.690882\t7.996300\t-0.397975\t-0.687807\t165.867170\t0.325000\t-0.052000\n\t\n15:41:00.4\tlog_raw\tgps_raw\t\tsystem status\tnormal 2 27.900000 0 0\trobot status\t210.502416\t111.731004\t7.996100\t-0.393409\t-0.661310\t165.824859\t0.248000\t0.068000\n\t\n15:41:00.9\tlog_raw\tgps_raw\t\tsystem status\tnormal 2 27.900000 0 0\trobot status\t210.368099\t111.773375\t7.995400\t-0.498349\t-0.727775\t165.841037\t0.377000\t-0.109000\n\t\n15:41:01.4\tlog_raw\tgps_raw\t#INSPVAXA,USB3,0,48.0,FINESTEERING,2107,283279.400,02000000,471d,15824;INS_ALIGNMENT_COMPLETE,INS_RTKFIXED,37.37113775239,126.72320841739,7.9941,22.3000,0.0997,-0.2552,-0.0140,-0.507226746,-0.753730833,284.120099148,0.4481,0.2971,0.5694,0.1142,0.0928,0.0780,0.0969,0.1021,4.9040,0f000001,0*1d440196\n\tsystem status\tnormal 2 27.900000 0 0\trobot status\t210.224116\t111.820545\t7.994100\t-0.507227\t-0.753731\t165.879901\t0.250000\t0.056000\n\t\n15:41:01.9\tlog_raw\tgps_raw\t\tsystem status\tnormal 2 27.900000 0 0\trobot status\t210.100141\t111.859831\t7.993400\t-0.665050\t-1.038178\t165.832812\t0.272000\t0.032000\n\t\n15:41:02.4\tlog_raw\tgps_raw\t\tsystem status\tnormal 2 27.900000 0 0\trobot status\t209.964462\t111.905154\t7.993800\t-0.597748\t-1.139572\t165.849053\t0.383000\t-0.124000\n\t\n15:41:02.9\tlog_raw\tgps_raw\t\tsystem status\tnormal 2 27.900000 0 0\trobot status\t209.830279\t111.950559\t7.993400\t-0.543948\t-1.065924\t165.832474\t0.273000\t0.052000\n\t\n15:41:03.4\tlog_raw\tgps_raw\t#INSPVAXA,USB3,0,49.5,FINESTEERING,2107,283281.400,02000000,471d,15824;INS_ALIGNMENT_COMPLETE,INS_RTKFIXED,37.37113937207,126.72320229897,7.9921,22.3000,0.0832,-0.2611,-0.0143,-0.573096548,-0.909868573,284.165048220,0.4480,0.2971,0.5695,0.1141,0.0928,0.0780,0.0969,0.1020,4.9063,0f000001,0*a447e184\n\tsystem status\tnormal 2 27.900000 0 0\trobot status\t209.682156\t112.000318\t7.992100\t-0.573097\t-0.909869\t165.834952\t0.279000\t0.027000\n\t\n15:41:03.9\tlog_raw\tgps_raw\t\tsystem status\tnormal 2 27.900000 0 0\trobot status\t209.557703\t112.041610\t7.991700\t-0.607082\t-0.999301\t165.784999\t0.248000\t0.073000\n\t\n15:41:04.4\tlog_raw\tgps_raw\t#INSPVAXA,USB3,0,46.5,FINESTEERING,2107,283282.400,02000000,471d,15824;INS_ALIGNMENT_COMPLETE,INS_RTKFIXED,37.37114019228,126.72319922313,7.9923,22.3000,0.0951,-0.2773,-0.0041,-0.536108170,-0.972919730,284.196085514,0.4479,0.2971,0.5695,0.1142,0.0928,
